vi "Ferma pompa auto.vi"() -> ()   [LabVIEW 2019]
panel:
  out "mod auto stop pompa?":bool
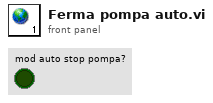
[diagram p1: front panel]
diagram:
